vi "Fluke 6105A Set.vi"(1 "Reset? (T: Yes)":bool=TRUE, 2 "Voltage or Current":enum16{"Voltage", "Current"}(ring), 4 "Phases":dbl[](array[numeric]), 5 "Upper Range":dbl=50.0, 6 "Amplitudes":dbl[](array[numeric]), 7 "Lower Range":dbl=20.0, 8 "Harmonics":i32[](array[numeric]), 9 "Enable Harmonics?":bool=TRUE, 10 "Frequency":i32=50, 11 "VISA resource name":refnum<visa-resource-name>="6105A") -> (0 "error out":errorcluster, 3 "VISA resource name out":refnum<visa-resource-name>)   [LabVIEW 2014]
doc: "This VI is a simple example showing how to configure global settings and 2 harmonics."
uses:
  SharedVariables/TSE_Variables.vi
panel:
  in  "Current Bandwidth":string(combo)="NORM"
  in  "Output Selector":u16(ring)=1 items=["L1"=1, "L2"=2, "L3"=3, "N"=4]
  in  "Sense Setting (1:4-wire)":u16(ring)=1 items=["2-wire sensing", "4-wire sensing"]
  in  "Angle Setting (0: Degrees)":string(combo)="DEG"
  in  "Line Locking (F: Off)":bool
  in  "stop":bool
  # "(c) 2004 - 2010 National Instruments.  ALL RIGHTS RESERVED."
  # "Global Settings"
  # "Voltage Harmonics Amplitude"
  # "Absolute RMS"
  # "Voltage Harmonics Amplitude"
  # "Absolute RMS"
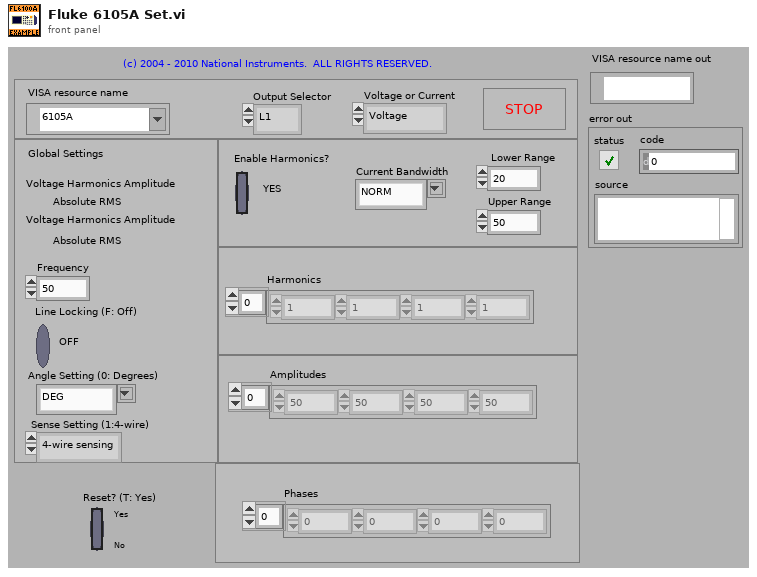
[diagram p1: front panel]
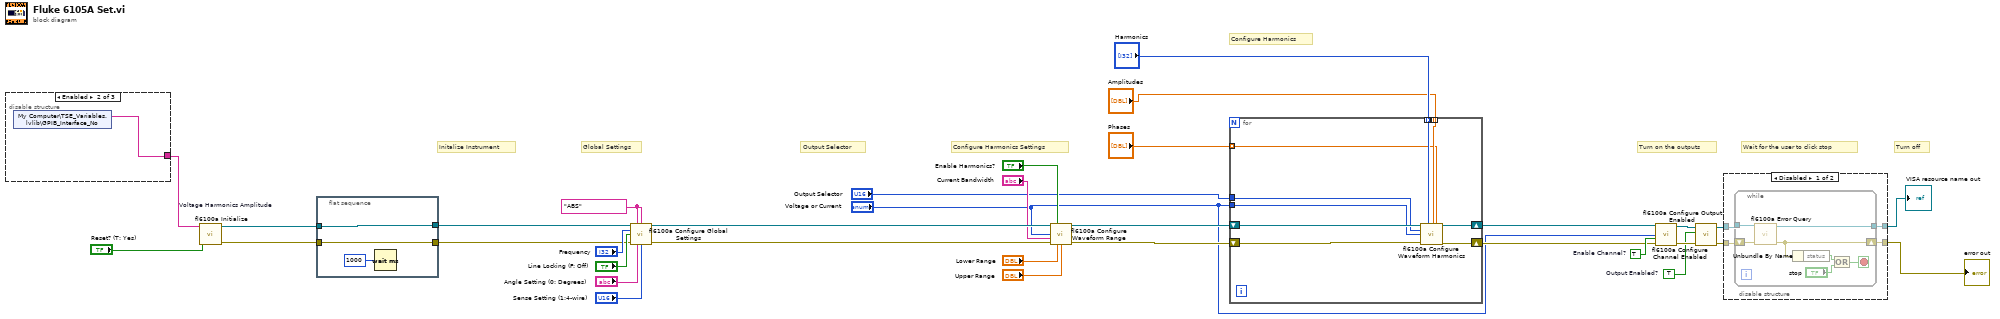
[diagram p0: block diagram]
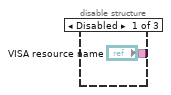
[diagram p2: hidden frame]
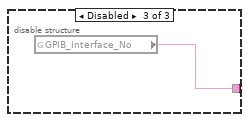
[diagram p3: hidden frame]
diagram:
  w17 = "ABS"  # Voltage Harmonics Amplitude
  w18 = TRUE  # Enable Channel?
  w19 = TRUE  # Output Enabled?
  # "Configure Harmonics"
  # "Turn off"
  # "Turn on the outputs"
  # "Wait for the user to click stop"
  # "Configure Harmonics Settings"
  # "Output Selector"
  # "Global Settings"
  # "Initalize Instrument"
  n1 = disable-structure shown="Enabled" {
    disable-tunnel: ["VISA resource name" w36 w37] -> w34
    frame Disabled {
    }
    frame Enabled {
      n2 = shared-variable "My Computer\\TSE_Variables.lvlib\\GPIB_Interface_No"() -> (w36:string)  [unwired: 1 in, 1 out]
    }
    frame Disabled {
      n3 = global read "TSE_Variables.vi" "GPIB_Interface_No"() -> (w37:string)
    }
  }
  n4 = call <instrlib>:"fl6100a Initialize.vi"("Reset? (T: Yes)"="Reset? (T: Yes)", "VISA resource name"=w34) -> ("error out"=w1:errorcluster, "VISA resource name out"=w3:refnum<visa-resource-name>)  [unwired: 8 in]
  n5 = flat-sequence {
    tunnel: [w40] -> w4
    tunnel: w3 -> [w40]
    tunnel: [w39] -> w2
    tunnel: w1 -> [w39]
    frame #0 {
      n6 = Wait (ms)(milliseconds to wait=u32 1000) -> ()  [unwired: 1 out]
    }
  }
  n7 = call <instrlib>:"fl6100a Configure Global Settings.vi"("VISA resource name"=w4, "Voltage Harmonics Amplitude (0: Absolute RMS)"=w17, "Current Harmonics Amplitude (0: Absolute RMS)"=w17, "Frequency (60 Hz)"="Frequency", "Line Locking (F: Off)"="Line Locking (F: Off)", "error in (no error)"=w2, "Angle Setting (0: Degrees)"="Angle Setting (0: Degrees)", "Sense Setting (1:4-wire)"="Sense Setting (1:4-wire)") -> ("VISA resource name out"=w29:refnum<visa-resource-name>, "error out"=w28:errorcluster)  [unwired: 6 in]
  n8 = call <instrlib>:"fl6100a Configure Waveform Range.vi"("VISA resource name"=w29, "Enable Harmonics? (F:NO)"="Enable Harmonics?", "Voltage or Current (0: Voltage)"="Voltage or Current", "Current Bandwidth (1:6000 Hz)"="Current Bandwidth", "error in (no error)"=w28, "Lower Range (1)"="Lower Range", "Upper Range (2)"="Upper Range") -> ("VISA resource name out"=w27:refnum<visa-resource-name>, "error out"=w26:errorcluster)  [unwired: 7 in]
  n9 = for {
    tunnel: "Output Selector" -> [w47]
    tunnel: "Voltage or Current" -> [w46]
    shift-right: [w45] -> w12
    shift-left: w27 -> [w49]
    shift-right: [w44] -> w11
    shift-left: w26 -> [w48]
    tunnel: "Harmonics" -> [w43] mode=indexing
    tunnel: "Amplitudes" -> [w42] mode=indexing
    tunnel: "Phases" -> [w41] mode=indexing
    n10 = call <instrlib>:"fl6100a Configure Waveform Harmonics.vi"("VISA resource name"=w49, "Harmonic (1)"=w43, "Amplitude (1)"=w42, "Phase Angle (0)"=w41, "Output Selector (0:L1)"=w47, "Voltage or Current (0: Voltage)"=w46, "error in (no error)"=w48) -> ("VISA resource name out"=w45:refnum<visa-resource-name>, "error out"=w44:errorcluster)  [unwired: 7 in]
  }
  n11 = call <instrlib>:"fl6100a Configure Channel Enabled.vi"("VISA resource name"=w12, "Voltage or Current (0: Voltage)"="Voltage or Current", "Enable Channel? (F:NO)"=w18, "error in (no error)"=w11) -> ("VISA resource name out"=w23:refnum<visa-resource-name>, "error out"=w20:errorcluster)  [unwired: 10 in]
  n12 = call <instrlib>:"fl6100a Configure Output Enabled.vi"("error in (no error)"=w20, "Enable Output? (F:NO)"=w19, "VISA resource name"=w23) -> ("error out"=w21:errorcluster, "VISA resource name out"=w22:refnum<visa-resource-name>)  [unwired: 7 in]
  n13 = disable-structure shown="Disabled" {
    disable-tunnel: w22 -> [w53 w62]
    disable-tunnel: w21 -> [w52 w61]
    disable-tunnel: [w51 w62] -> w14
    disable-tunnel: [w50 w61] -> w13
    frame Disabled {
      n14 = while {
        tunnel: w53 -> [w60]
        shift-right: [w58] -> w50
        shift-left: w52 -> [w59]
        tunnel: [w54] -> w51
        stop <- w55 stop-if-true
        n15 = call <instrlib>:"fl6100a Error Query.vi"("error in (no error)"=w59, "VISA resource name"=w60) -> ("error out"=w58:errorcluster, "VISA resource name out"=w54:refnum<visa-resource-name>)  [unwired: 6 in, 2 out]
        n16 = Unbundle By Name(w58) -> ("status"=w57:bool)
        n17 = Or(x=w57, y="stop") -> (x .or. y?=w55:bool)
      }
    }
    frame Enabled {
    }
  }
  "VISA resource name out" <- w14
  "error out" <- w13
